vi "Append Carriage Return Character.vi"(8 "error in (no error)":errorcluster, 10 "Command":string) -> (0 "error out":errorcluster, 2 "Command Out":string)   [LabVIEW 2011, in "Roboteq.lvlib"]
doc: "Appends a carriage return character to the command."
uses:
  Roboteq.lvlib
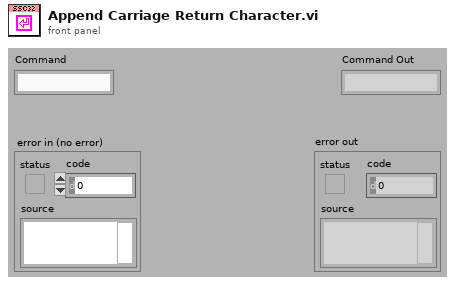
[diagram p1: front panel]
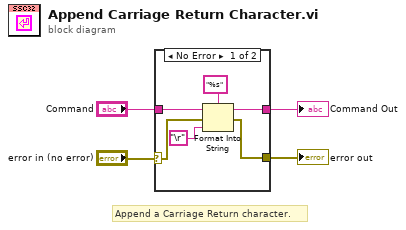
[diagram p0: block diagram]
diagram:
  # "Append a Carriage Return character."
  n1 = case shown="No Error" "error in (no error)" {
    selector: "error in (no error)" -> [w7 w11]
    tunnel: "Command" -> [w10 _]
    tunnel: [w6 _] -> w1
    tunnel: [w5 w11] -> w2
    frame No Error {
      n2 = Format Into String(format string="%s", initial string=w10, error in=w7, "\r") -> (resulting string=w6:string, error out=w5:errorcluster)
    }
    frame Error {
    }
  }
  "Command Out" <- w1
  "error out" <- w2
